vi "Tacho2Velocity_params.vi"(0 "Action (Read)":T3=enum."Read", 2 "Tachometer param input":T1={"Offset [V]"=0.0, "Gain [deg/sV]"=130.0}, 3 "ETH Mike Model":T2) -> (5 "Cluster":T1={"Offset [V]"=0.0, "Gain [deg/sV]"=130.0})   [LabVIEW 2019]
uses:
  ReadOnlyGlobalActions.ctl
  ETHMikeModel.ctl
  TypeDefTachometerParam.ctl
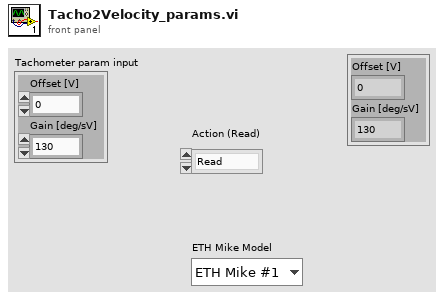
[diagram p1: front panel]
types:
  T1 = typedef "TypeDefTachometerParam.ctl" = cluster{"Offset [V]":dbl, "Gain [deg/sV]":dbl}
  T2 = typedef "ETHMikeModel.ctl" = enum16{"ETH Mike #1", "ETH Mike #2", "ETH Mike #3", "ETH Mike #4", "ETH MIKE #5", "ETH Mike #6"}
  T3 = typedef "ReadOnlyGlobalActions.ctl" = enum16{"Initialize", "Read", "Write"}
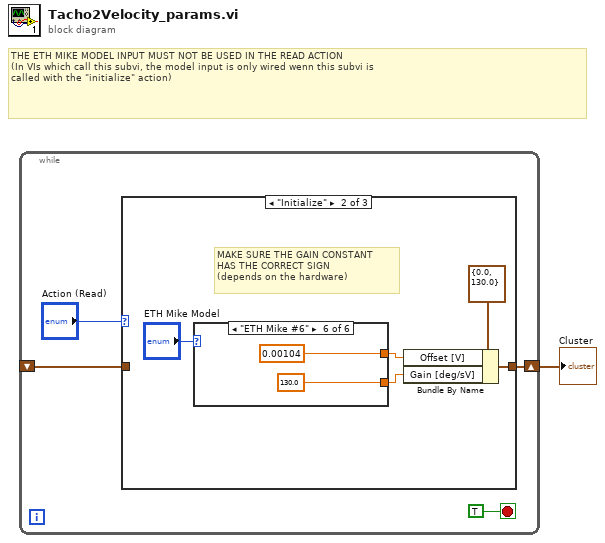
[diagram p0: block diagram]
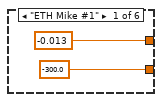
[diagram p3: hidden frame]
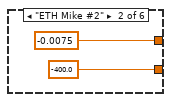
[diagram p4: hidden frame]
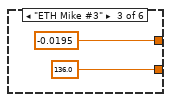
[diagram p5: hidden frame]
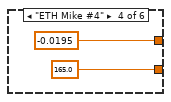
[diagram p6: hidden frame]
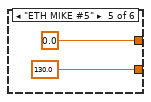
[diagram p7: hidden frame]
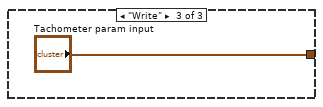
[diagram p8: hidden frame]
diagram:
  # "THE ETH MIKE MODEL INPUT MUST NOT BE USED IN THE READ ACTION\n(In VIs which call this subvi, the model input is only wired wenn this subvi is\ncalled with the \"initialize\" action)"
  n1 = while {
    shift-right: [w4] -> w1
    shift-left: _ -> [w3]
    stop <- TRUE stop-if-true
    n2 = case shown="\"Initialize\"" "Action (Read)" {
      tunnel: [w6 w9 "Tachometer param input"] -> w4
      tunnel: w3 -> [w6 _ _]
      frame "Read" {
      }
      frame "Initialize" {
        # "MAKE SURE THE GAIN CONSTANT\nHAS THE CORRECT SIGN \n(depends on the hardware)"
        n3 = case shown="\"ETH Mike #6\"" "ETH Mike Model" {
          tunnel: [-0.013 ("Offset [V]") -0.0075 ("Offset [V]") -0.0195 ("Offset [V]") -0.0195 ("Offset [V]") 0.0 ("Offset [V]") 0.00104 ("Offset [V]")] -> w7
          tunnel: [-300.0 ("Gain [deg/sV]") -400.0 ("Gain [deg/sV]") 136.0 ("Gain [deg/sV]") 165.0 ("Gain [deg/sV]") 130.0 ("Gain [deg/sV]") 130.0 ("Gain [deg/sV]")] -> w8
          frame "ETH Mike #1" {
          }
          frame "ETH Mike #2" {
          }
          frame "ETH Mike #3" {
          }
          frame "ETH Mike #4" {
          }
          frame "ETH MIKE #5" {
          }
          frame "ETH Mike #6" {
          }
        }
        n4 = Bundle By Name(cluster=T1 {"Offset [V]"=0.0, "Gain [deg/sV]"=130.0}, "Offset [V]"=w7, "Gain [deg/sV]"=w8) -> (w9:T1)
      }
      frame "Write" {
      }
    }
  }
  "Cluster" <- w1
